vi "Frequency Measurements - Large Range with 2 Counters.vi"() -> ()   [LabVIEW 2009]
uses:
  <vilib>/DAQmx/create/channels.llb/DAQmx Create Channel (CI-Frequency).vi
  <vilib>/DAQmx/read.llb/DAQmx Read (Counter DBL 1Chan 1Samp).vi
panel:
  in  "divisor":u32=4
  in  "stop":bool
  in  "counter":tag
  out "Frequency (Hz)":dbl format="%0.2f"
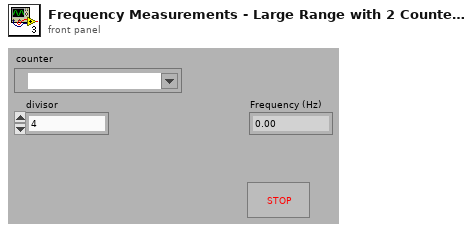
[diagram p1: front panel]
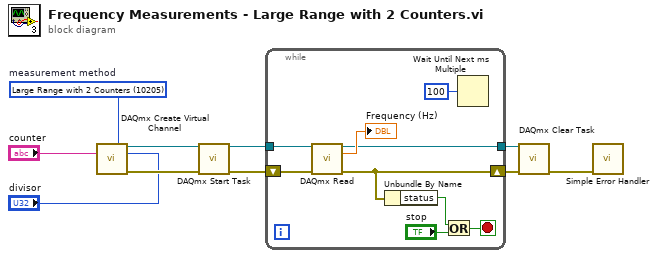
[diagram p0: block diagram]
diagram:
  w9 = 10205 items=["Low Frequency with 1 Counter"=10105, "High Frequency with 2 Counters"=10157, "Large Range with 2 Counters"=10205]  # measurement method
  n1 = call-poly <vilib>:"DAQmx Create Virtual Channel.vi"("measurement method"=w9, "counter"="counter", "divisor"="divisor") -> ("task out"=w8:refnum<k21>, "error out"=w6:errorcluster)  [unwired: 11 in]
  n2 = call <vilib>:"DAQmx Start Task.vi"("task/channels in"=w8, "error in"=w6) -> ("task out"=w7:refnum<k21>, "error out"=w5:errorcluster)  [unwired: 12 in]
  n3 = while {
    tunnel: w7 -> [w17]
    shift-right: [w16] -> w3
    shift-left: w5 -> [w18]
    tunnel: [w11] -> w4
    stop <- w15 stop-if-true
    n4 = call-poly <vilib>:"DAQmx Read.vi"("task/channels in"=w17, "error in"=w18) -> ("task out"=w11:refnum<k21>, "data"=→"Frequency (Hz)":dbl, "error out"=w16:errorcluster)  [unwired: 11 in]
    n5 = Unbundle By Name "Unbundle By Name"(w16) -> ("status"=w14:bool)
    n6 = Or(x=w14, y="stop") -> (x .or. y?=w15:bool)
    n7 = Wait Until Next ms Multiple(millisecond multiple=u32 100) -> ()  [unwired: 1 out]
  }
  n8 = call <vilib>:"DAQmx Clear Task.vi"("task in"=w4, "error in"=w3) -> ("error out"=w2:errorcluster)  [unwired: 13 in]
  n9 = call <vilib>:"Simple Error Handler.vi"("error in (no error)"=w2) -> ()  [unwired: 4 in, 5 out]
